vi "Ctor.vi"(8 "error in (no error)":errorcluster, 11 "Device in":refnum<class "Device.lvclass">) -> (0 "error out":errorcluster, 3 "Device out":refnum<class "Device.lvclass">)   [LabVIEW 2020, in "HAL.lvlib" / "Device.lvclass"]
uses:
  Device.lvclass
  Ref Data.ctl
  Device State.ctl
  Device.lvclass/Device.ctl
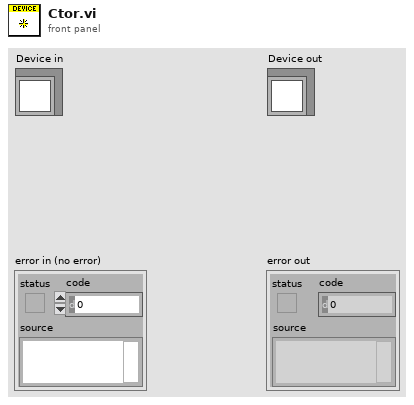
[diagram p1: front panel]
types:
  T1 = typedef "HAL.lvlib/Device.lvclass/Device State.ctl" = enum16{"Uninitialized", "Initialized", "Configured", "Running", "Error"}
  T2 = typedef "HAL.lvlib/Device.lvclass/Ref Data.ctl" = cluster{"Config Keys":string[], "Config Values":string[], "Cal Expires":timestamp, "Name":string, "Comment":string, "State":T1, "Error":errorcluster}
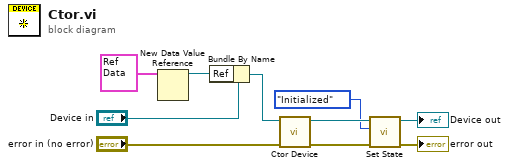
[diagram p0: block diagram]
diagram:
  n1 = New Data Value Reference(data value=T2 {"Config Keys"=[], "Config Values"=[], "Cal Expires"=timestamp(0 s since 1904-01-01), "Name"="", "Comment"="", "State"=enum."Uninitialized", "Error"={"status"=FALSE, "code"=0, "source"=""}} ("Ref Data")) -> (data value reference=w8:refnum<data-value>)  [unwired: 1 in, 1 out]
  n2 = Bundle By Name(cluster="Device in", "Ref"=w8) -> (w6:refnum<class "Device.lvclass">)
  n3 = call-dynamic "Ctor Device.vi"("error in (no error)"="error in (no error)", "Device in"=w6) -> ("error out"=w5:errorcluster, "Device out"=w4:refnum<class "Device.lvclass">)  [unwired: 8 in]
  n4 = call "Set State.vi"("error in (no error)"=w5, "Device State"=Device_State."Initialized", "Device in"=w4) -> ("error out"=→"error out":errorcluster, "Device out"=→"Device out":refnum<class "Device.lvclass">)  [unwired: 7 in]
